vi "remote_control.vi"() -> (3 "Final X, Y, BEARING":cluster{dbl, dbl, dbl})   [LabVIEW 2017]
uses:
  <vilib>/myRIO/Common/Instrument Driver Framework/myRIO v1.0/Encoder/typedefs/Encoder Signal Mode.ctl
  <vilib>/myRIO/Instrument Drivers/Onboard IO/Encoder/typedefs/Encoder Reference.ctl
  <vilib>/myRIO/Common/Instrument Driver Framework/Utilities/typedefs/myRIO Generic Hardware Reference.ctl
  <vilib>/myRIO/Common/Instrument Driver Framework/Utilities/typedefs/Hardware Version Enum.ctl
  <vilib>/myRIO/Common/Instrument Driver Framework/Utilities/typedefs/myRIO v1.0 Reference.ctl
  <vilib>/myRIO/Common/Instrument Driver Framework/Utilities/typedefs/Generic FPGA Reference.ctl
  <vilib>/myRIO/Common/Instrument Driver Framework/myRIO v1.0/Encoder/typedefs/Encoder Channels Enum.ctl
  <vilib>/myRIO/Common/Instrument Driver Framework/myRIO v1.0/Encoder/typedefs/Encoder Configuration v1.0.ctl
  <vilib>/userdefined/High Color/nirio_resource_hc.ctl
  <vilib>/myRIO/Common/Instrument Driver Framework/Utilities/vis/Is FPGA Ref Available.vi
  <vilib>/myRIO/Common/Instrument Driver Framework/myRIO v1.0/Encoder/vis/myRIO v1.1 Open Encoder.vi
  <vilib>/myRIO/Instrument Drivers/Onboard IO/Encoder/vis/Read.vi
  <vilib>/myRIO/Common/Instrument Driver Framework/Utilities/vis/Validate Channels.vi
  <vilib>/myRIO/Common/Instrument Driver Framework/myRIO v1.0/Encoder/vis/myRIO v1.0 Reserve Encoder.vi
  <vilib>/myRIO/Common/Instrument Driver Framework/myRIO v1.0/Encoder/vis/myRIO v1.0 Build MUX Configuration Encoder.vi
  <vilib>/myRIO/Common/Instrument Driver Framework/myRIO v1.0/Resource Manager/vis/myRIO v1.0 Reserve Channel List.vi
  <vilib>/myRIO/Common/Instrument Driver Framework/myRIO v1.0/Resource Manager/vis/myRIO v1.0 Create Configuration List.vi
  <vilib>/myRIO/Common/Instrument Driver Framework/myRIO v1.0/Resource Manager/vis/myRIO v1.0 Reserve Channel.vi
  <vilib>/myRIO/Common/Instrument Driver Framework/myRIO v1.0/Resource Manager/vis/myRIO v1.0 Unreserve Channel.vi
  <vilib>/myRIO/Common/Instrument Driver Framework/myRIO v1.0/Resource Manager/vis/myRIO v1.0 Build Mutex Name.vi
  <vilib>/Utility/VariantDataType/GetNumericInfo.vi
  <vilib>/Utility/error.llb/Error Cluster From Error Code.vi
  <vilib>/myRIO/Common/Instrument Driver Framework/myRIO v1.0/myRIO v1.1 Open.vi
  <vilib>/myRIO/Common/Instrument Driver Framework/Utilities/vis/IO Manager.vi
  <vilib>/myRIO/Common/Instrument Driver Framework/Utilities/vis/Configuration Manager.vi
  <vilib>/myRIO/Common/Instrument Driver Framework/myRIO v1.0/Resource Manager/vis/myRIO v1.0 Configure IO.vi
  <vilib>/myRIO/Common/Instrument Driver Framework/myRIO v1.0/myRIO v1.0 Close.vi
  <vilib>/myRIO/Common/Instrument Driver Framework/myRIO v1.0/Encoder/vis/myRIO v1.0 Configure Encoder.vi
  <vilib>/myRIO/Common/Instrument Driver Framework/myRIO v1.0/Encoder/vis/myRIO v1.0 Read Encoder.vi
  <vilib>/addons/control/pid/pid.llb/PID (DBL).vi
  <vilib>/myRIO/Express VI/Onboard IO/Encoder/Encoder Express VI.xnode
  <vilib>/myRIO/Instrument Drivers/Onboard IO/Encoder/vis/myRIO Encoder Open.xnode
  <vilib>/myRIO/Common/Instrument Driver Framework/myRIO v1.0/Encoder/typedefs/Encoder Count Direction Enum.ctl
  <vilib>/addons/control/pid/NI_PID_pid.lvlib
  <vilib>/myRIO/Instrument Drivers/Onboard IO/Encoder/Encoder.lvlib
  <vilib>/Analysis/NI_AALPro.lvlib
  <vilib>/robotics/Navigation/shared/WorldMap/OccupancyGridWorldMap/NI_Robotics_OccupancyGridWorldMap.lvclass
panel:
  out "XY Graph 2":cluster{dbl[], dbl[]}(graph)
  in  "stop 2":bool
  in  "Resolution":dbl=50.0
  out "Intensity Graph":dbl[][](graph)
  out "Frequency":u32=10
  in  "curPos":cluster{"x":i32, "y":i32}
  in  "endPos":cluster{"x":i32, "y":i32}={"x"=0, "y"=6}
  out "path":cluster{"X":i32, "Y":i32}[](array[cluster])
  out "X, Y, BEARING 2":cluster{dbl, dbl, dbl}
  in  "Speed":dbl(slide) scale=-10.0..10.0
  in  "Angle":dbl(slide) scale=-360.0..360.0
  out "XY Graph":cluster{"X":dbl, "Y":dbl}[](graph)=[{"X"=3.638988671509065, "Y"=989.3451951487937}, {"X"=3.4680482195157727, "Y"=989.91873657972}]
  in  "PID gains":T1={"proportional gain (Kc)"=0.05, "integral time (Ti, min)"=0.05, "derivative time (Td, min)"=0.0} {"derivative time (Td, min)" format="%.3f"; "integral time (Ti, min)" format="%.3f"; "proportional gain (Kc)" format="%.3f"}
  in  "stop":bool
  out "OUTPUT B":dbl(slide)=1.4 scale=-10.0..10.0
  out "OUTPUT A":dbl(slide)=0.7407999999999447 scale=-10.0..10.0
  out "PID A":T2(graph)={"Setpoint"=0.6006479088049201, "output"=0.05446764760463431, "dx/dt"=0.7407999999999447}
  out "PID B":T2(graph)={"Setpoint"=1.3993520911950799, "output"=0.10115092019020398, "dx/dt"=1.4}
  out "Setpoint A":dbl(slide)=0.6006479088049201 scale=-10.0..10.0
  out "Setpoint B":dbl(slide)=1.3993520911950799 scale=-10.0..10.0
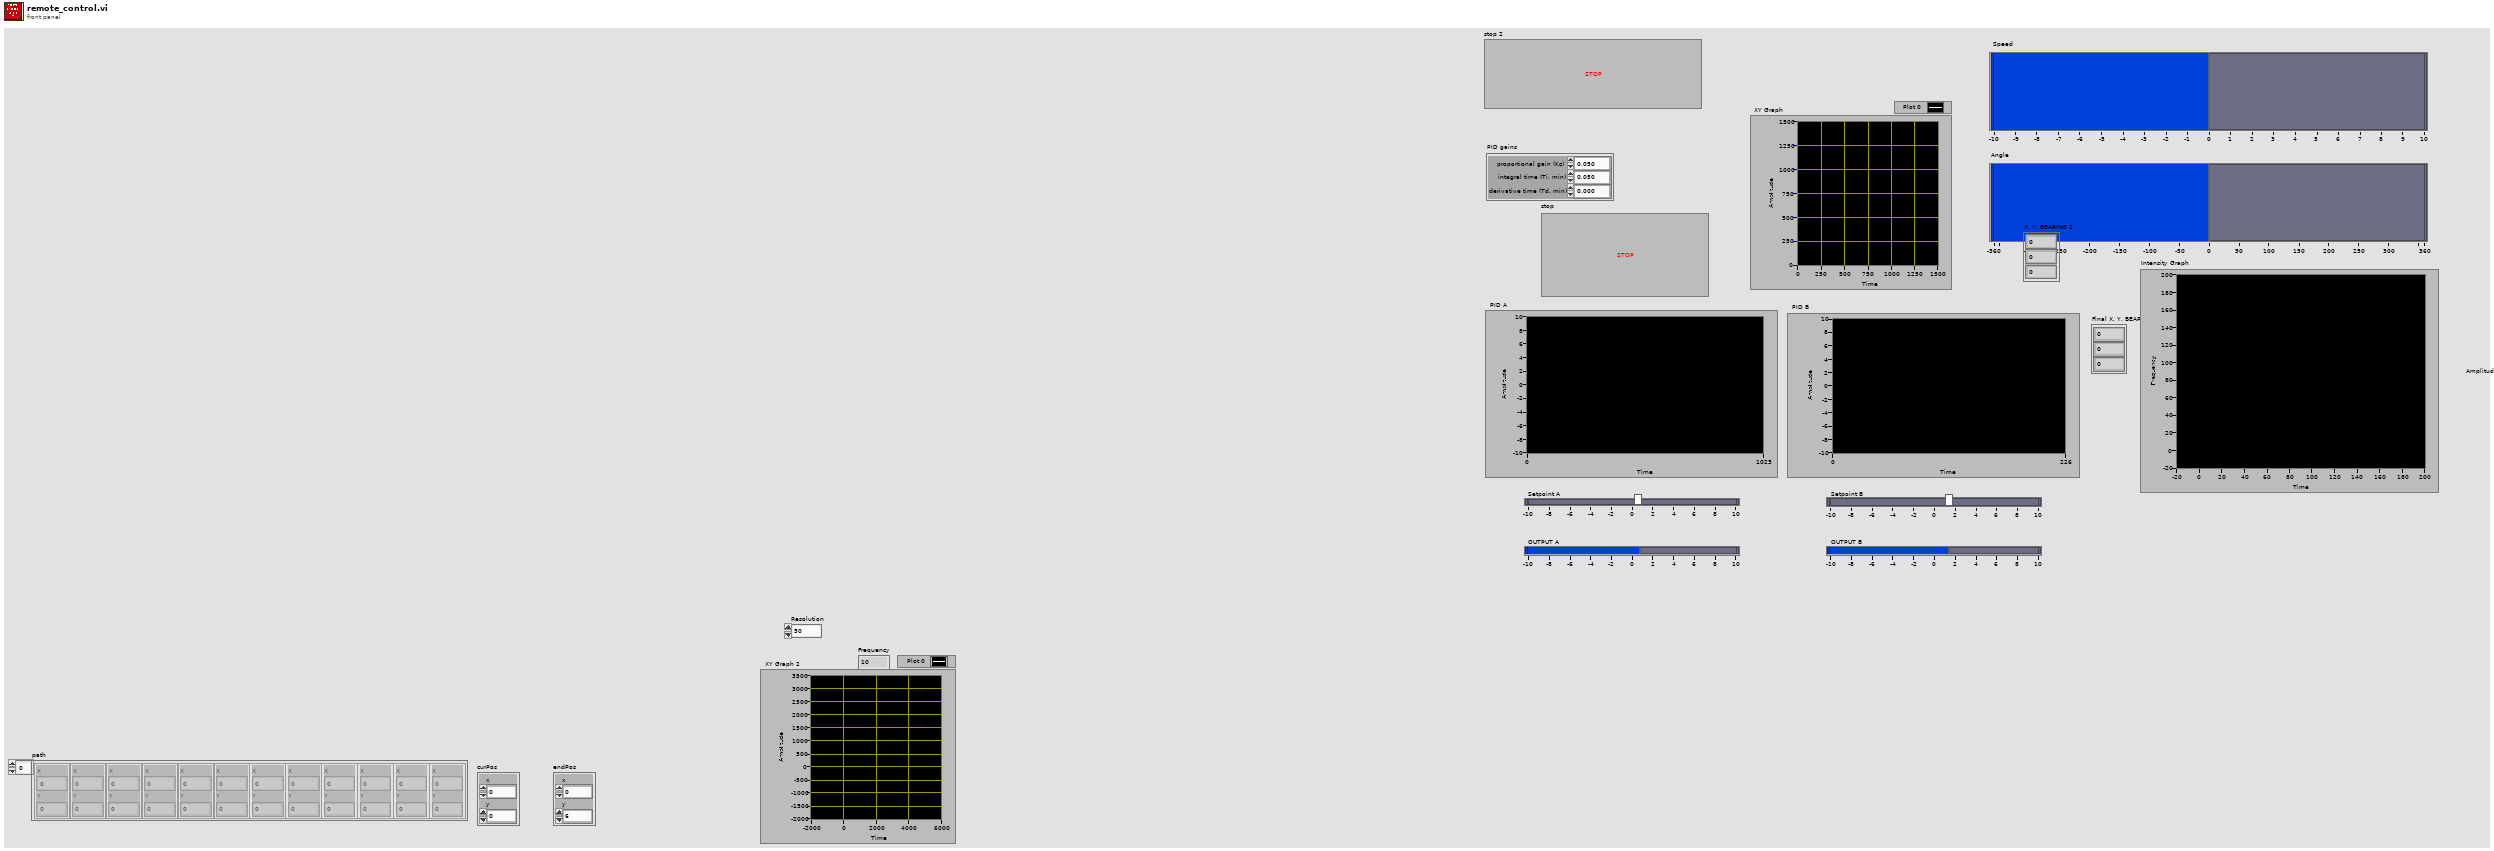
[diagram p1: front panel]
types:
  T1 = cluster{"proportional gain (Kc)":dbl, "integral time (Ti, min)":dbl, "derivative time (Td, min)":dbl}
  T2 = cluster{"Setpoint":dbl, "output":dbl, "dx/dt":dbl}
  T3 = typedef "LidarPoint.ctl" = cluster{"X":dbl, "Y":dbl}
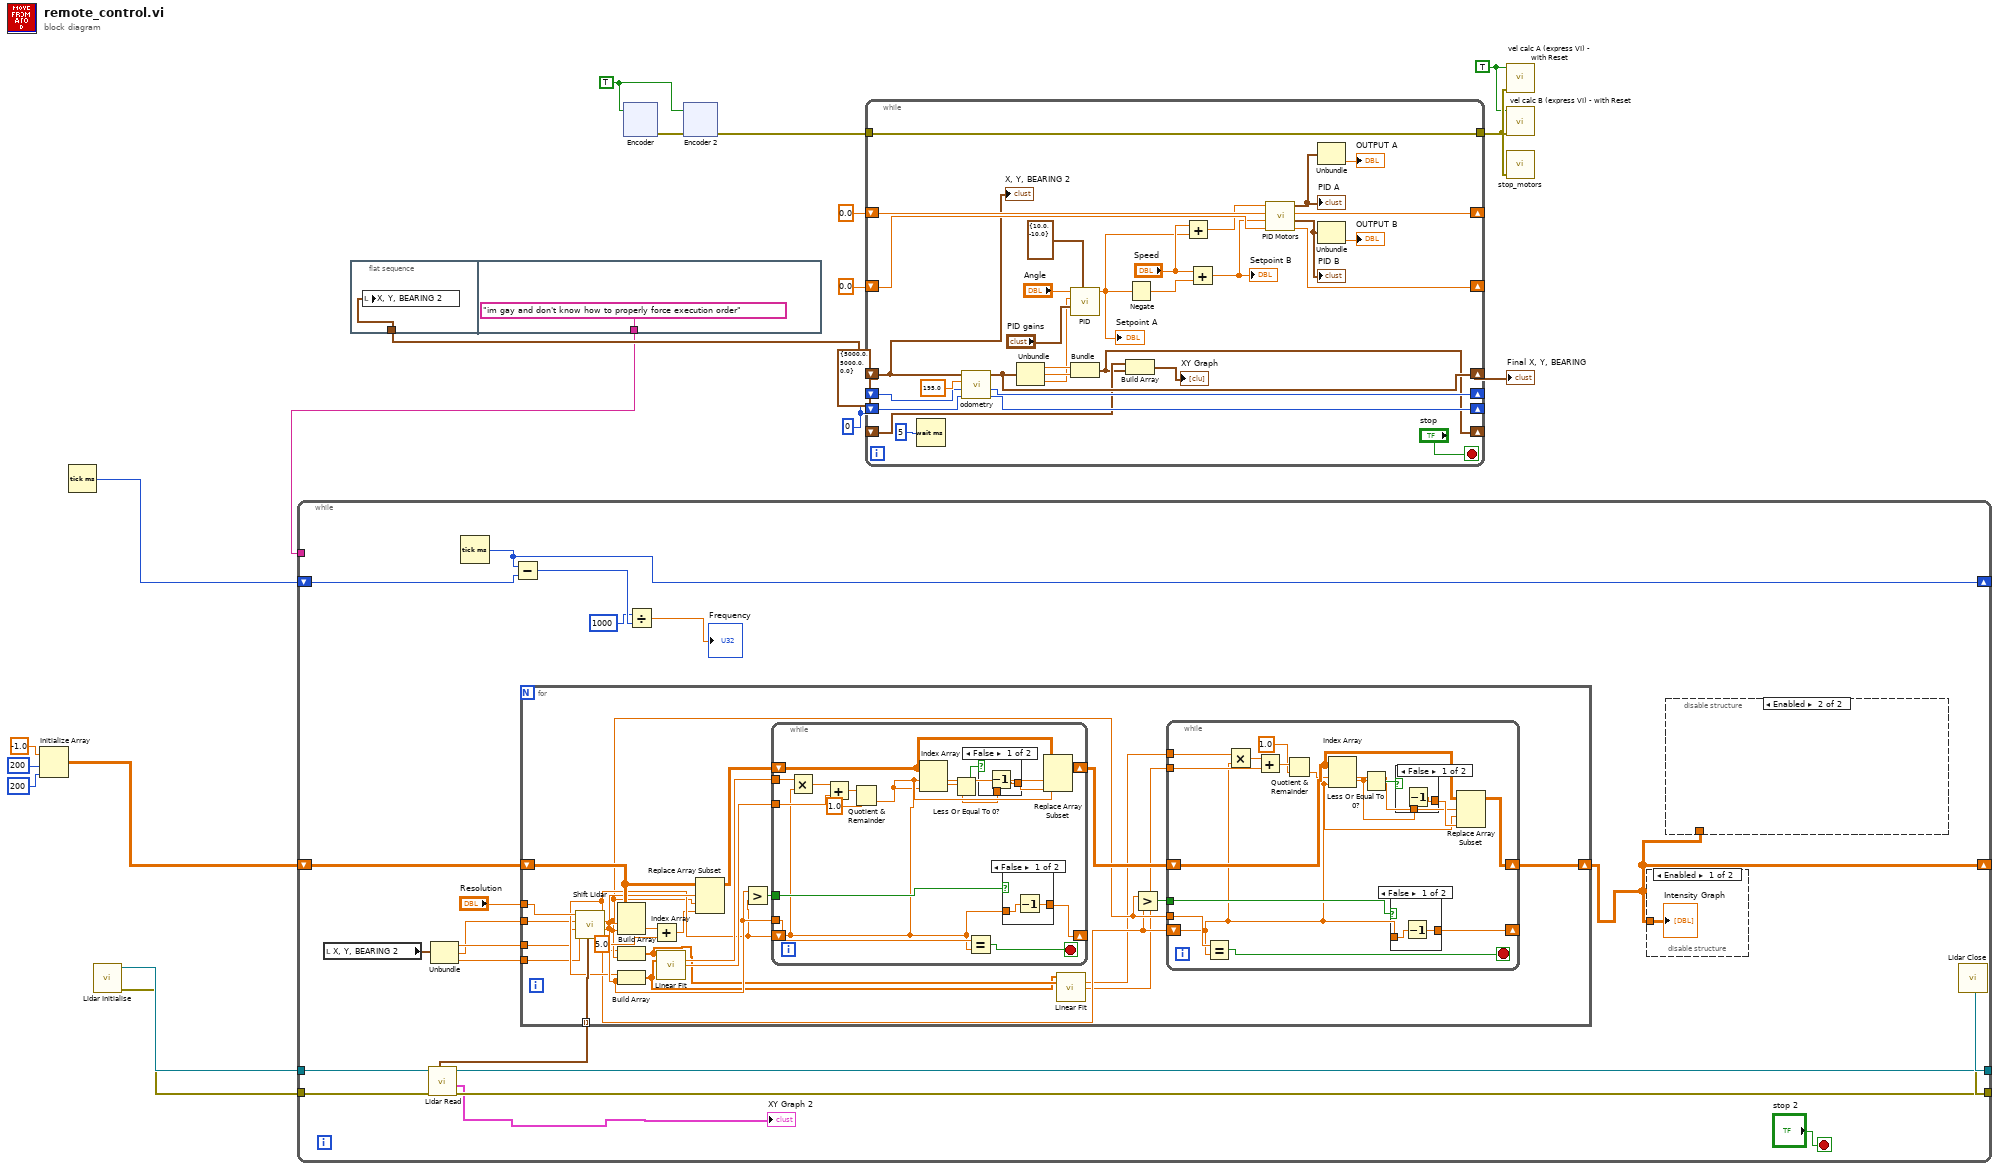
[diagram p0: block diagram]
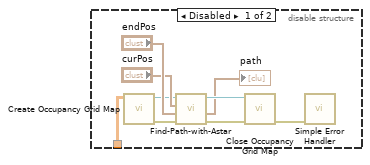
[diagram p2: hidden frame]
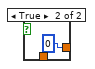
[diagram p4: hidden frame]
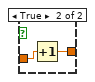
[diagram p5: hidden frame]
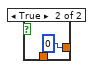
[diagram p6: hidden frame]
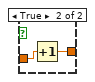
[diagram p7: hidden frame]
diagram:
  w2 = cluster{dbl, dbl, dbl} {5000.0, 5000.0, 0.0} ("Initial X, Y, BEARING")
  w12 = TRUE ("Reinitialise")
  w14 = TRUE
  w16 = 0 ("ENCA OUT")
  n1 = Initialize Array(-1.0 ("element"), 200 ("dimension size"), 200 ("dimension size")) -> (w5:dbl[][])
  n2 = Tick Count (ms)() -> (millisecond timer value=w3:u32)
  n3 = call "Lidar Initialise.vi"() -> ("error out"=w10:errorcluster, "VISA resource name out"=w11:refnum<visa-resource-name>)  [unwired: 10 in]
  n4 = while {
    tunnel: w11 -> [w39]
    tunnel: w10 -> [w38]
    tunnel: [w37] -> w9
    tunnel: [w36] -> w8
    shift-right: [w27] -> _
    shift-left: w5 -> [w33]
    shift-right: [w30] -> _
    shift-left: w3 -> [w32]
    tunnel: w1 -> [_]
    stop <- "stop 2" stop-if-true
    n5 = local read "X, Y, BEARING 2"() -> (w24:cluster{dbl, dbl, dbl})
    n6 = call "Lidar Read.vi"("error in (no error)"=w38, "VISA resource name"=w39) -> ("error out"=w36:errorcluster, "Visual Out"=→"XY Graph 2":cluster{dbl[], dbl[]}, "VISA resource name out"=w37:refnum<visa-resource-name>, "XYflipped"=w25:T3[])  [unwired: 2 in, 3 out]
    n7 = Unbundle(w24) -> (w23:dbl, w22:dbl, w21:dbl)
    n8 = Tick Count (ms)() -> (millisecond timer value=w30:u32)
    n9 = Subtract(x=w30, y=w32) -> (x-y=w29:u32)
    n10 = for {
      tunnel: "Resolution" -> [w73]
      tunnel: w25 -> [w72] mode=indexing
      shift-right: [w60] -> w27
      shift-left: w33 -> [w71]
      tunnel: w23 -> [w52]
      tunnel: w22 -> [w51]
      tunnel: w21 -> [w50]
      n11 = call "Shift Lidar.vi"("XY"=w72, "Angle"=w50, "X position"=w52, "Y position"=w51, "Resolution"=w73) -> ("PosY"=w58:dbl, "Shifted X"=w68:dbl, "Shifted Y"=w59:dbl, "PosX"=w65:dbl)  [unwired: 3 in]
      n12 = Index Array(array=w71, index (row)=w68, index (col)=w59) -> (element=w64:dbl)
      n13 = Build Array(w58, w59) -> (w56:dbl[])
      n14 = Build Array(w65, w68) -> (w55:dbl[])
      n15 = Add(x=w64, y=5.0) -> (x+y=w63:dbl)
      n16 = call <vilib>:"Linear Fit.vi"("Y"=w56, "X"=w55) -> ("slope"=w70:dbl, "intercept"=w69:dbl)  [unwired: 9 in, 3 out]
      n17 = Replace Array Subset(array=w71, new element=w63, index (row)=w68, index (col)=w59) -> (w66:dbl[][])
      n18 = Greater?(x=w68, y=w65) -> (0:w67:bool)
      n19 = while {
        tunnel: w68 -> [w111]
        shift-right: [w109] -> _
        shift-left: w65 -> [w104]
        tunnel: w70 -> [w108]
        tunnel: w69 -> [w106]
        tunnel: w67 -> [w110]
        shift-right: [w103] -> w61
        shift-left: w66 -> [w105]
        stop <- w112 stop-if-true
        n20 = Multiply(x=w108, y=w104) -> (x*y=w107:dbl)
        n21 = Add(x=w107, y=w106) -> (x+y=w99:dbl)
        n22 = Quotient & Remainder(x=w99, y=1.0) -> (floor(x/y)=w97:dbl)  [unwired: 1 out]
        n23 = Index Array(array=w105, index (row)=w104, index (col)=w97) -> (element=w100:dbl)
        n24 = Less Or Equal To 0?(x=w100) -> (x <= 0?=w102:bool)
        n25 = Equal?(x=w111, y=w104) -> (x = y?=w112:bool)
        n26 = case shown="False" w102 {
          tunnel: [w114 0] -> w101
          tunnel: w100 -> [w113 _]
          frame False {
            n27 = Decrement(x=w113) -> (x-1=w114:dbl)
          }
          frame True {
          }
        }
        n28 = case shown="False" w110 {
          tunnel: w104 -> [w116 w119]
          tunnel: [w117 w118] -> w109
          frame False {
            n29 = Decrement(x=w116) -> (x-1=w117:dbl)
          }
          frame True {
            n30 = Increment(x=w119) -> (x+1=w118:dbl)
          }
        }
        n31 = Replace Array Subset(array=w105, new element=w101, index (row)=w104, index (col)=w97) -> (w103:dbl[][])
      }
      n32 = call <vilib>:"Linear Fit.vi"("Y"=w55, "X"=w56) -> ("slope"=w54:dbl, "intercept"=w53:dbl)  [unwired: 9 in, 3 out]
      n33 = Greater?(x=w59, y=w58) -> (0:w57:bool)
      n34 = while {
        shift-right: [w78] -> w60
        shift-left: w61 -> [w77]
        shift-right: [w86] -> _
        shift-left: w58 -> [w75]
        tunnel: w59 -> [w88]
        tunnel: w57 -> [w87]
        tunnel: w54 -> [w85]
        tunnel: w53 -> [w83]
        stop <- w89 stop-if-true
        n35 = Equal?(x=w88, y=w75) -> (x = y?=w89:bool)
        n36 = Multiply(x=w85, y=w75) -> (x*y=w84:dbl)
        n37 = Add(x=w84, y=w83) -> (x+y=w82:dbl)
        n38 = Quotient & Remainder(x=w82, y=1.0) -> (floor(x/y)=w74:dbl)  [unwired: 1 out]
        n39 = Index Array(array=w77, index (row)=w74, index (col)=w75) -> (element=w79:dbl)
        n40 = Less Or Equal To 0?(x=w79) -> (x <= 0?=w80:bool)
        n41 = case shown="False" w87 {
          tunnel: w75 -> [w93 w96]
          tunnel: [w94 w95] -> w86
          frame False {
            n42 = Decrement(x=w93) -> (x-1=w94:dbl)
          }
          frame True {
            n43 = Increment(x=w96) -> (x+1=w95:dbl)
          }
        }
        n44 = case shown="False" w80 {
          tunnel: [w91 0] -> w76
          tunnel: w79 -> [w90 _]
          frame False {
            n45 = Decrement(x=w90) -> (x-1=w91:dbl)
          }
          frame True {
          }
        }
        n46 = Replace Array Subset(array=w77, new element=w76, index (row)=w74, index (col)=w75) -> (w78:dbl[][])
      }
    }
    n47 = Divide(x=u32 1000 ("y"), y=w29) -> (x/y=→"Frequency":dbl)
    n48 = disable-structure shown="Enabled" {
      disable-tunnel: w27 -> [w49 _]
      frame Enabled {
        "Intensity Graph" <- w49
      }
      frame Disabled {
      }
    }
    n49 = disable-structure shown="Enabled" {
      disable-tunnel: w27 -> [w40 _]
      frame Disabled {
        n50 = call <vilib>:"Create Occupancy Grid Map.vi"("occupancy grid"=w40) -> ("error out"=w48:errorcluster, "map reference out"=w45:refnum<data-value>)  [unwired: 9 in]
        n51 = call "Find-Path-with-Astar.vi"("error in (no error)"=w48, "goal node"="endPos", "start node"="curPos", "map reference in"=w45) -> ("error out"=w43:errorcluster, "Array"=→"path":cluster{"X":i32, "Y":i32}[], "map reference out"=w44:refnum<data-value>)  [unwired: 5 in]
        n52 = call <vilib>:"Close Occupancy Grid Map.vi"("error in (no error)"=w43, "map reference in"=w44) -> ("error out"=w42:errorcluster)  [unwired: 9 in]
        n53 = call <vilib>:"Simple Error Handler.vi"("error in (no error)"=w42) -> ()  [unwired: 4 in, 5 out]
      }
      frame Enabled {
      }
    }
  }
  n54 = flat-sequence {
    tunnel: w2 -> [w120]
    tunnel: ["im gay and don't know how to properly force execution order"] -> w1
    frame #0 {
      n55 = local write "X, Y, BEARING 2"(w120) -> ()
    }
    frame #1 {
    }
  }
  n56 = xnode "Encoder"("Reset Counter"=w14) -> ("error out"=w15:errorcluster)  [unwired: 1 in, 3 out]
  n57 = xnode "Encoder 2"("error in (no error)"=w15, "Reset Counter"=w14) -> ("error out"=w13:errorcluster)  [unwired: 3 out]
  n58 = while {
    tunnel: w13 -> [w148]
    shift-right: [w150] -> _
    shift-left: 0.0 ("output A") -> [w151]
    shift-right: [w152] -> _
    shift-left: 0.0 ("output B") -> [w127]
    tunnel: [w148] -> w19
    shift-right: [w140] -> _
    shift-left: w16 -> [w142]
    shift-right: [w139] -> _
    shift-left: w16 -> [w141]
    shift-right: [w138] -> w20
    shift-left: w2 -> [w122]
    shift-right: [w134] -> _
    shift-left: _ -> [w135]
    stop <- "stop" stop-if-true
    n59 = Wait (ms)(milliseconds to wait=5 ("ENCB OUT")) -> ()  [unwired: 1 out]
    n60 = call "odometry.vi"("ENCB in"=w141, "ENCA in"=w142, "wheelbase"=195.0, "Position"=w122) -> ("ENCB OUT"=w139:i32, "ENCA OUT"=w140:i32, "X, Y, BEARING"=w138:cluster{dbl, dbl, dbl})  [unwired: 4 in]
    n61 = Unbundle(w138) -> (w136:dbl, w137:dbl, w131:dbl)
    n62 = call-poly <vilib>:"PID.vi"("output range"=cluster{"output high":dbl, "output low":dbl} {"output high"=10.0, "output low"=-10.0}, "PID gains"="PID gains", "process variable"=w131, "setpoint"="Angle") -> ("output"=w124:dbl)  [unwired: 6 in, 1 out]
    "Setpoint A" <- w124
    n63 = Bundle(w136, w137) -> (w134:cluster{dbl, dbl})  [unwired: 1 in]
    n64 = Build Array(w135, w134) -> (→"XY Graph":cluster{dbl, dbl}[])
    n65 = Negate(x=w124) -> (-x=w125:dbl)
    n66 = Add(x="Speed", y=w124) -> (x+y=w123:dbl)
    n67 = Add(x="Speed", y=w125) -> (x+y=w126:dbl)
    "Setpoint B" <- w126
    n68 = call "PID Motors.vi"("input B"=w127, "Speed B"=w126, "input A"=w151, "Speed A"=w123) -> ("output B"=w152:dbl, "Speed B0"=w146:T2, "output A"=w150:dbl, "Speed A0"=w147:T2)
    "PID B" <- w146
    "PID A" <- w147
    n69 = Unbundle(w147) -> ("dx/dt"=→"OUTPUT A":dbl)  [unwired: 2 out]
    n70 = Unbundle(w146) -> ("dx/dt"=→"OUTPUT B":dbl)  [unwired: 2 out]
    "X, Y, BEARING 2" <- w122
  }
  "Final X, Y, BEARING" <- w20
  n71 = call "vel calc A (express VI) - with Reset.vi"("error in"=w19, "Reinitialise"=w12) -> ()  [unwired: 5 in, 5 out]
  n72 = call "vel calc B (express VI) - with Reset.vi"("error in"=w19, "Reinitialise"=w12) -> ()  [unwired: 5 in, 5 out]
  n73 = call "stop_motors.vi"("error in (no error)"=w19) -> ()  [unwired: 4 in, 1 out]
  n74 = call "Lidar Close.vi"("error in (no error)"=w8, "VISA resource name"=w9) -> ()  [unwired: 9 in, 1 out]
